vi "MC5e Build_Unit_Listbox.vi"(8 "error in (no error)":errorcluster, 11 "Unit Multilist Ref":refnum<vi>) -> (0 "error out":errorcluster)   [LabVIEW 2020]
uses:
  MC5e Unit.ctl
  MC5e Terrain types.ctl
  MC5e Squad_Info.ctl
  MC5e Size_Categories.ctl
  MC5e Unit Header.ctl
  Location.ctl
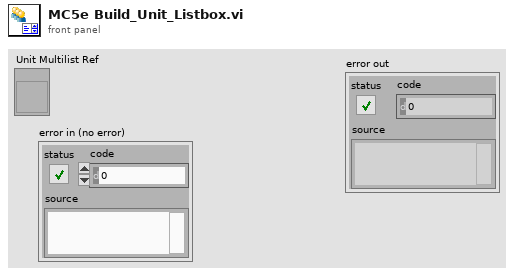
[diagram p1: front panel]
types:
  T1 = typedef "MC5e Unit.ctl" = cluster{"Unit Fatigue Level":enum16{"Not Fatigued", "Fatigued", "Seriously Fatigued"}, "Flying Unit":bool, "Mounted Unit":bool, "Defending from Stronghold":bool, "Difficult Terrain Types":T2, "Squads in Unit":T3[], "Unit Info":T5, "Range":i32, "BR":i32, "Speed":i32, "Morale":i32, "Current BR":i32, "Location":T6, "Capacity %":i32}
  T2 = typedef "MC5e Terrain types.ctl" = i32[]
  T3 = typedef "MC5e Squad_Info.ctl" = cluster{"Squad Name":string, "# Soldiers":u16, "Battle Rating":u16, "Flying":bool, "Mounted":bool, "Speed":u16, "Range":u16, "Morale":i32, "Max Endurance":u16, "Current Endurance":i32, "Size":T4, "Space Taken":u16, "Difficult Terrain":i32[], "CR":u16, "Special / Notes":string}
  T4 = typedef "MC5e Size_Categories.ctl" = enum16{"Tiny", "Small", "Medium", "Large", "Huge", "Gargantuan"}
  T5 = typedef "MC5e Unit Header.ctl" = cluster{"Unit Name":string, "Unit Commander":string, "Morale Mod":i32, "BR Mod":i32, "Defense Mod":i32, "Speed Mod":i32, "Unit Notes":string, "Attack Mod":i32, "Unit Wins+ Losses-":i32, "Commander Charisma Bonus":i32}
  T6 = typedef "Location.ctl" = cluster{"X coordinate":dbl, "Y coordinate":dbl}
  T7 = enum16{"Not Fatigued", "Fatigued", "Seriously Fatigued"}
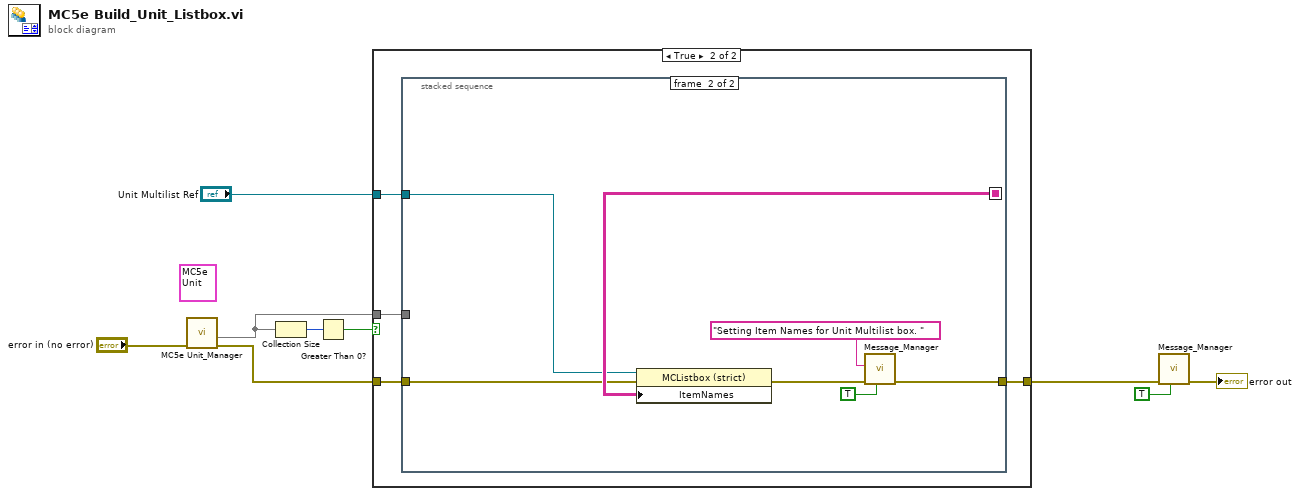
[diagram p0: block diagram]
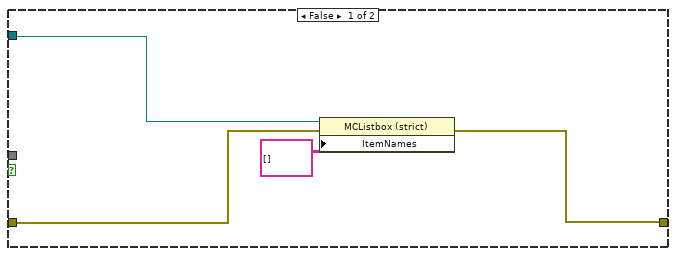
[diagram p2: hidden frame]
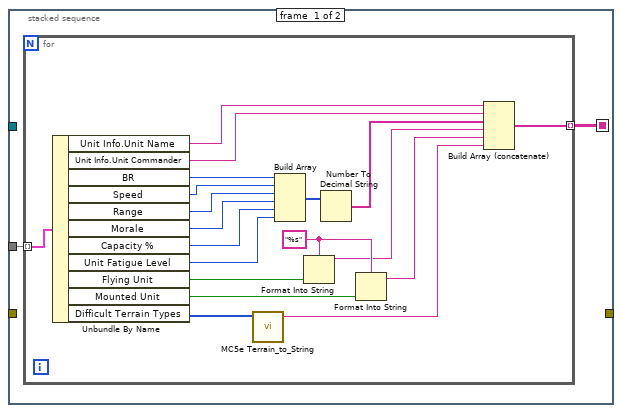
[diagram p3: hidden frame]
diagram:
  (unwired) T1 {"Unit Fatigue Level"=enum."Not Fatigued", "Flying Unit"=FALSE, "Mounted Unit"=FALSE, "Defending from Stronghold"=FALSE, "Difficult Terrain Types"=[0, 1, 3, 6, 7], "Squads in Unit"=[], "Unit Info"={"Unit Name"="", "Unit Commander"="", "Morale Mod"=0, "BR Mod"=0, "Defense Mod"=0, "Speed Mod"=0, "Unit Notes"="", "Attack Mod"=0, "Unit Wins+ Losses-"=0, "Commander Charisma Bonus"=0}, "Range"=0, "BR"=0, "Speed"=0, "Morale"=0, "Current BR"=0, "Location"={"X coordinate"=0.0, "Y coordinate"=0.0}, "Capacity %"=0} ("Unit In (Add/Replace)")
  n1 = call "MC5e Unit_Manager.vi"("error in"="error in (no error)") -> ("error out"=w3:errorcluster, "Set Out"=w2:set{T1})  [unwired: 7 in, 2 out]
  n2 = Collection Size(1:w2) -> (0:w9:i32)
  n3 = Greater Than 0?(x=w9) -> (x > 0?=w8:bool)
  n4 = case shown="True" w8 {
    tunnel: w3 -> [w11 w17]
    tunnel: w2 -> [_ w16]
    tunnel: [w10 w15] -> w6
    tunnel: "Unit Multilist Ref" -> [w12 w14]
    frame False {
      n5 = property class="MCListbox (strict)"(reference=w12, error in=w11, "ItemNames"=string[][] [] ("Item Names")) -> (error out=w10:errorcluster)  [unwired: 1 out]
    }
    frame True {
      n6 = stacked-sequence {
        seq-local: [w18 _] -> [_ w45]
        tunnel: w17 -> [_ w44]
        tunnel: w16 -> [w19 _]
        tunnel: [_ w40] -> w15
        tunnel: w14 -> [_ w43]
        frame #0 {
          n7 = for {
            tunnel: w19 -> [w38] mode=indexing
            tunnel: [w37] -> w18 mode=indexing
            w23 = "%s" ("format string")
            n8 = Unbundle By Name(w38) -> ("Unit Info.Unit Name"=w36:string, "Unit Info.Unit Commander"=w27:string, "BR"=w34:i32, "Speed"=w33:i32, "Range"=w32:i32, "Morale"=w31:i32, "Capacity %"=w30:i32, "Unit Fatigue Level"=w29:T7, "Flying Unit"=w25:bool, "Mounted Unit"=w24:bool, "Difficult Terrain Types"=w35:T2)
            n9 = call "MC5e Terrain_to_String.vi"("Difficult Terrain"=w35) -> ("Difficult Terrain String"=w20:string)  [unwired: 10 in]
            n10 = Build Array(w34, w33, w32, w31, w30, w29) -> (w28:i32[])
            n11 = Format Into String(format string=w23, w25) -> (resulting string=w22:string)  [unwired: 2 in, 1 out]
            n12 = Number To Decimal String(number=w28) -> (decimal integer string=w26:string[])  [unwired: 1 in]
            n13 = Format Into String(format string=w23, w24) -> (resulting string=w21:string)  [unwired: 2 in, 1 out]
            n14 = Build Array (concatenate)(w36, w27, w26, w22, w21, w20) -> (w37:string[])
          }
        }
        frame #1 {
          n15 = property class="MCListbox (strict)"(reference=w43, error in=w44, "ItemNames"=w45) -> (error out=w41:errorcluster)  [unwired: 1 out]
          n16 = call "Message_Manager.vi"("Log only on Err (F)"=TRUE ("Log only on Err"), "error in"=w41, "New Entry"="Setting Item Names for Unit Multilist box. ") -> ("error out"=w40:errorcluster)  [unwired: 4 in, 4 out]
        }
      }
    }
  }
  n17 = call "Message_Manager.vi"("Log only on Err (F)"=TRUE ("Log only on Err"), "error in"=w6) -> ("error out"=→"error out":errorcluster)  [unwired: 5 in, 4 out]
